vi "buildDataPaths_multiAxis.vi"(7 "Axis":i16(ring)=2 items=["x-axis", "y-axis"], 10 "expName":string="23-Mar-2016exp001_dataIn.csv", 11 "Data Folder":path=path "C:/Users/arnold/Documents/MATLAB/AFM_statespace/System Identification/data") -> (0 "dataOut path":path, 1 "metaData Path":path, 3 "dataIn Path":path)   [LabVIEW 2017]
panel:
  # "The point of this VI is to build paths for the DataIn.csv, dataOut.csv and metaData.csv\nbased off of the experiment name. I'm trying to come up with an easy way here..."
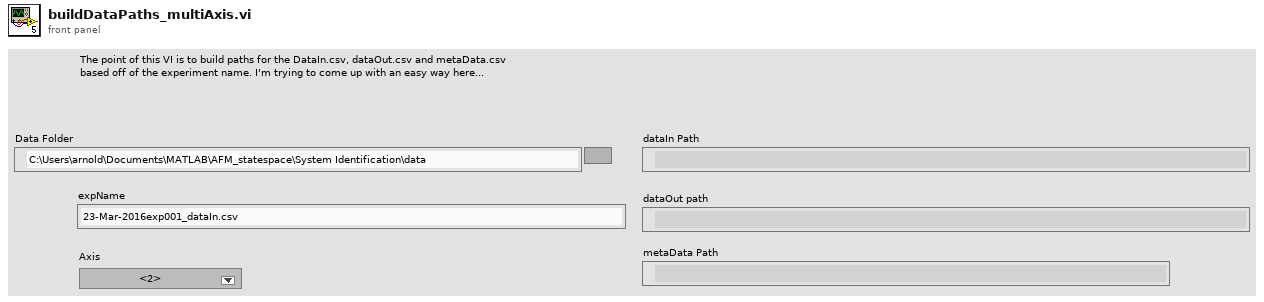
[diagram p1: front panel]
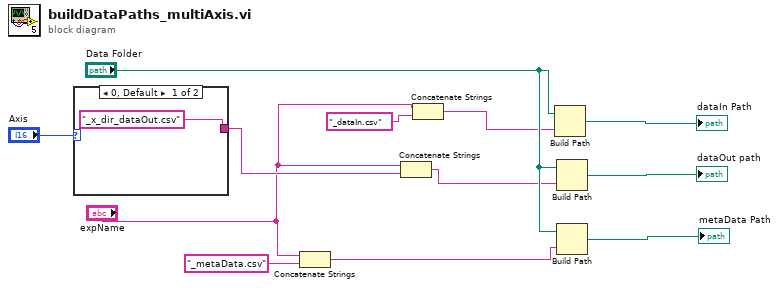
[diagram p0: block diagram]
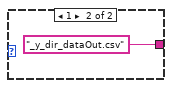
[diagram p2: hidden frame]
diagram:
  n1 = case shown="0, Default" "Axis" {
    tunnel: ["_x_dir_dataOut.csv" ("Data Out") "_y_dir_dataOut.csv" ("Data Out")] -> w5
    frame 0, Default {
    }
    frame 1 {
    }
  }
  n2 = Concatenate Strings("expName", "_metaData.csv" ("meta data name")) -> (w10:string)
  n3 = Concatenate Strings("expName", w5) -> (w2:string)
  n4 = Concatenate Strings("expName", "_dataIn.csv" ("input signals file")) -> (w1:string)
  n5 = Build Path(base path="Data Folder", name or relative path=w1) -> (appended path=→"dataIn Path":path)
  n6 = Build Path(base path="Data Folder", name or relative path=w2) -> (appended path=→"dataOut path":path)
  n7 = Build Path(base path="Data Folder", name or relative path=w10) -> (appended path=→"metaData Path":path)
